vi "Translator.Translate.Status (Single).vi"(8 "error in (no error)":errorcluster, 9 "Arg":variant, 10 "Msg":T1) -> (0 "error out":errorcluster, 2 "Translated Msg":string)   [LabVIEW 2019, in "Tools.lvlib"]
uses:
  Tools.lvlib
  Translator.Messages.Status.ctl
  <vilib>/dlg_ctls.llb/Space Constant.vi
  Translator.Global.vi
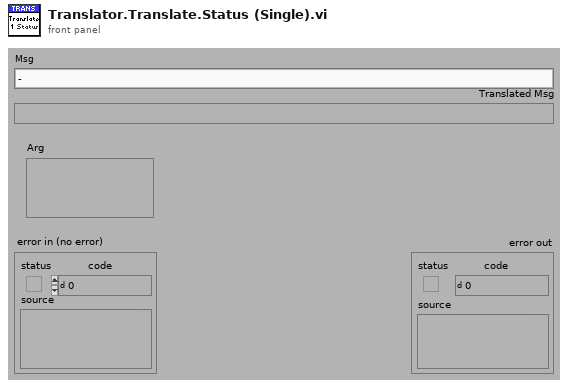
[diagram p1: front panel]
types:
  T1 = typedef "Tools.lvlib/Translator.Messages.Status.ctl" = enum16{"-", "Initializing...", "Quitting...", "Close the application?", "Log out?", "System", "All", "IDLE", "Translating...%s", "Restart is required to translate the application! Do you want to restart the PC?", "Restart cancelled. Be aware that some controls may not be fully translated until you restart the application.", "New version available!", "The software is up-to-date", "PC software will be updated after rebooting the PC. Do you want to reboot now?", "RT software will be updated. Make sure that no process is running. Do you want to reboot RT now?", "Updating RT firmware. Please wait...", "Update failed: %s", "Rebooting...", "Rebooting RT. Please wait...", "RT updated to version %s", "Timeout error during update. Check if RT is working", "Closing stations...", "Closing camera interface...", "Closing data acquisition interface...", "Service Option not available in this station!"}
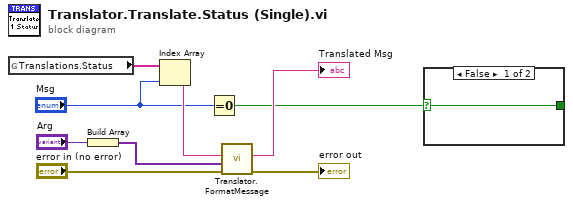
[diagram p0: block diagram]
diagram:
  n1 = global read "Translator.Global.vi" "Translations.Status"() -> (w7:string[])
  n2 = Build Array("Arg") -> (w3:variant[])
  n3 = Index Array(array=w7, index="Msg") -> (element=w6:string)
  n4 = Equal To 0?(x="Msg") -> (x = 0?=w1:bool)
  n5 = call "Translator.FormatMessage.vi"("error in (no error)"="error in (no error)", "Arguments"=w3, "Msg"=w6) -> ("error out"=→"error out":errorcluster, "Translated Msg"=→"Translated Msg":string)  [unwired: 7 in]
  n6 = case shown="False" w1 {
    selector: w1 -> [w10 w11]
    tunnel: [w10 w11] -> _
    frame False {
    }
    frame True {
    }
  }
